vi "Main - network stream.vi"(8 "error in (no error)":T1) -> (0 "error out":T1)   [LabVIEW 2019, in "Communication Interface.lvlib"]
uses:
  Communication Interface.lvlib
  Intertarget communication/Status + response + data cluster.ctl
  module state.ctl
  module data.ctl
  Intertarget communication/CR_master_class/CR_master.lvclass
  Intertarget communication/CR slave_class/CR slave.lvclass
  5bf6cc24-2521-4779-a80f-885c0f377251.vi
  Intertarget communication/NS slave_class/NS slave.lvclass
  C:/Barkhausen mmWave radar/Development/modules/mmw_instrument/src_LabVIEW/Host/Intertarget communication/CR slave_class/CR slave.lvclass
  Intertarget communication/UE_master_class/UE_master.lvclass
  C:/Barkhausen mmWave radar/Development/modules/mmw_instrument/src_LabVIEW/Host/Intertarget communication/CR_master_class/CR_master.lvclass
  SubVIs/Shared/Comm GV.vi
  SubVIs/Shared/System GV.vi
  Intertarget communication/CommandResponse communication.lvlib
  SubVIs/Shared/Shared.lvlib
  ZMQ_mmWave_class/ZMQ_mmWave.lvclass
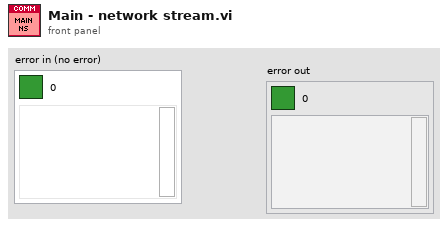
[diagram p1: front panel]
types:
  T1 = cluster{"Boolean Round":bool, "code":i32, "source":string}
  T2 = typedef "Communication Interface.lvlib/module state.ctl" = enum16{"init", "wait on connection", "communication", "close"}
  T3 = typedef "CommandResponse communication.lvlib/Status + response + data cluster.ctl" = cluster{"message":string, "response":string, "data":variant}
  T4 = typedef "Communication Interface.lvlib/module data.ctl" = cluster{"dummy":dbl, "HW Control":refnum<class "CR_master.lvclass">, "Command interface":refnum<class "CR slave.lvclass">}
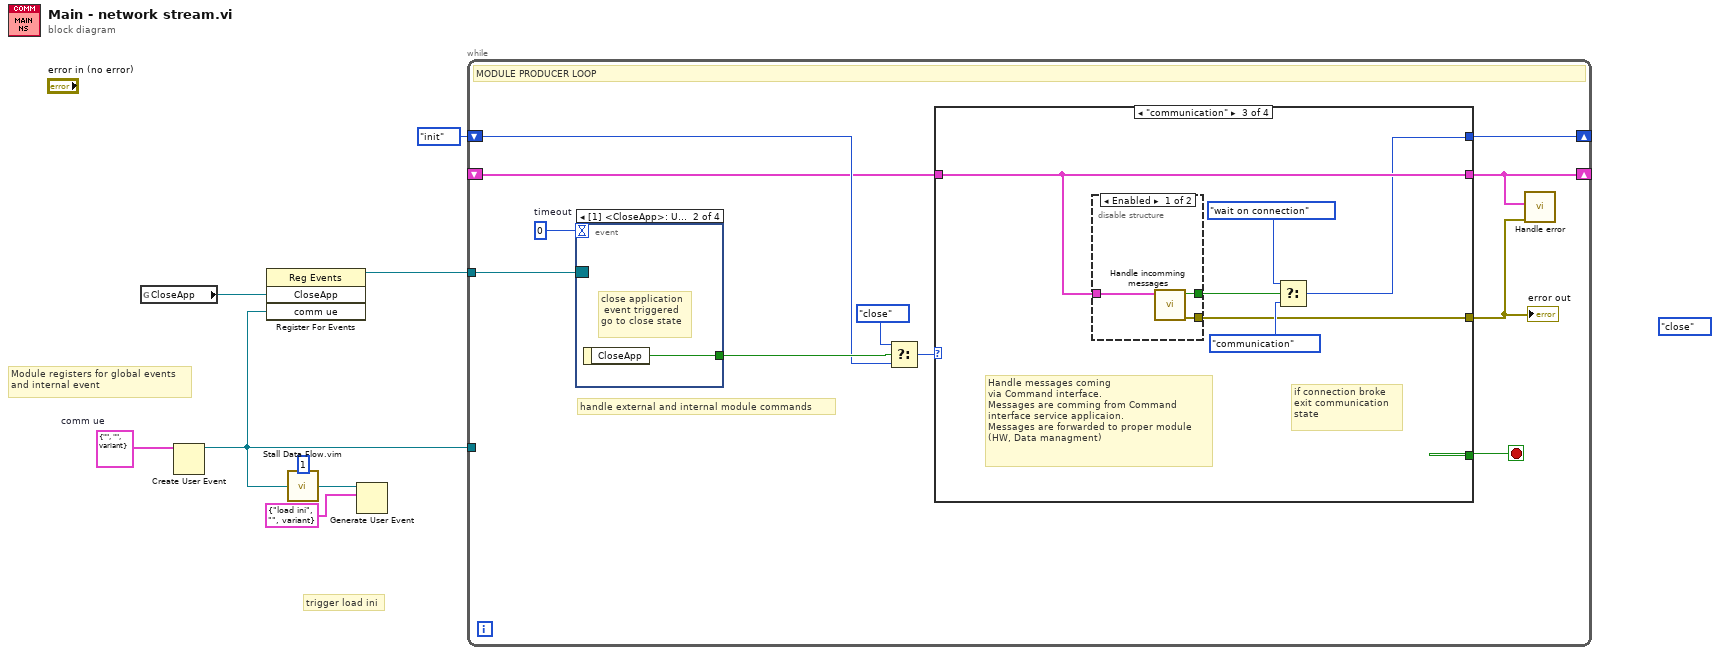
[diagram p0: block diagram]
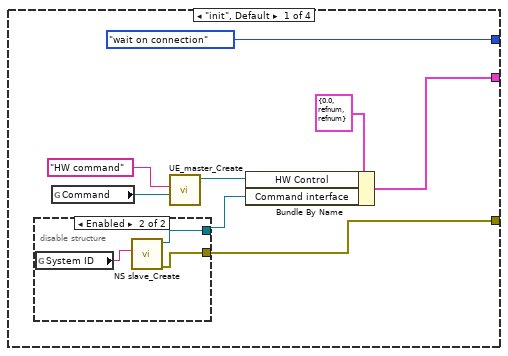
[diagram p2: hidden frame]
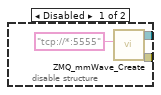
[diagram p3: hidden frame]
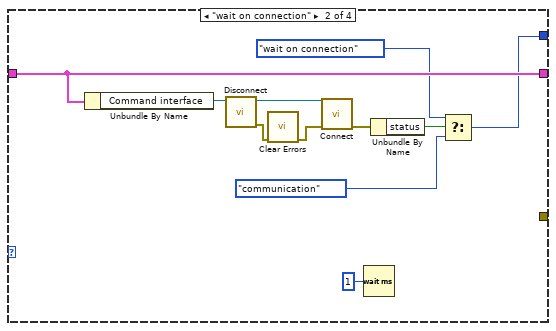
[diagram p4: hidden frame]
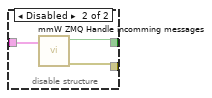
[diagram p5: hidden frame]
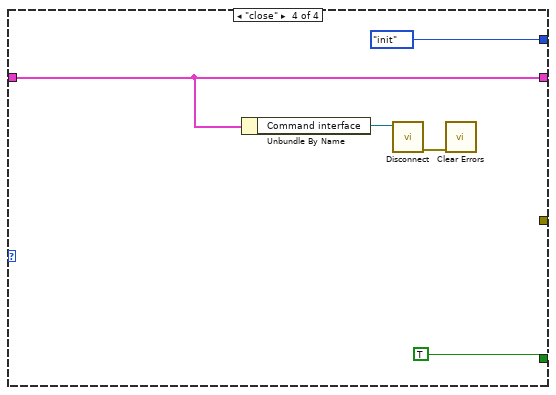
[diagram p6: hidden frame]
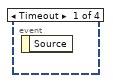
[diagram p7: hidden frame]
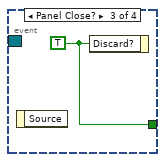
[diagram p8: hidden frame]
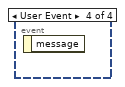
[diagram p9: hidden frame]
diagram:
  w4 = T3 {"message"="", "response"="", "data"=variant}  # comm ue
  (unwired) module_state."close" ("module states")
  # "trigger load ini"
  # "Module registers for global events\nand internal event"
  n1 = global read "Comm GV.vi" "CloseApp"() -> (w2:refnum<user-event>)
  n2 = Create User Event(user event datatype=w4) -> (user event=w7:refnum<user-event>)  [unwired: 1 in, 1 out]
  n3 = register-events(w2, w7) -> (reference out=w8:refnum<event-registration>)  [unwired: 2 in, 1 out]
  n4 = call "Stall Data Flow.vim"("value in"=w7, "milliseconds to wait"=u32 1) -> ("value out"=w6:refnum<user-event>)  [unwired: 1 out]
  n5 = Generate User Event(user event=w6, event data cluster=T3 {"message"="load ini", "response"="", "data"=variant} ("internal command")) -> ()  [unwired: 2 in, 2 out]
  n6 = while {
    tunnel: w8 -> [w19]
    tunnel: w7 -> [_]
    shift-right: [w11] -> _
    shift-left: _ -> [w12]
    shift-right: [w17] -> _
    shift-left: module_state."init" ("module states") -> [w15]
    stop <- w10 stop-if-true
    w18 = 0  # timeout
    # "handle external and internal module commands"
    # "MODULE PRODUCER LOOP"
    n7 = event shown="[1] <CloseApp>: User Event" {
      selector: w19 -> [_ _ _ _]
      dyn-events: _ -> [_ _ _ _]
      timeout: w18 -> [_ _ _ _]
      tunnel: [_ w62 w63 _] -> w16
      event Timeout {
        n8 = event-data() -> ()  [unwired: 1 in, 1 out]
      }
      event User Event {
        # "close application\n event triggered\ngo to close state"
        n9 = event-data() -> ("CloseApp"=w62:bool)  [unwired: 1 in]
      }
      event Panel Close? {
        w63 = TRUE ("Discard?")
        n10 = event-data() -> ()  [unwired: 1 in, 1 out]
        n11 = event-data("Discard?"=w63) -> ()  [unwired: 1 in, 1 out]
      }
      event User Event {
        n12 = event-data() -> ()  [unwired: 1 in, 1 out]
      }
    }
    n13 = Select(t=module_state."close", s=w16, f=w15) -> (s? t:f=w13:T2)
    n14 = case shown="\"communication\"" w13 {
      tunnel: [module_state."wait on connection" ("module states") w39 w47 module_state."init" ("t")] -> w17
      tunnel: [w21 w43 w50 w60] -> w11
      tunnel: w12 -> [_ w43 w50 w60]
      tunnel: [_ _ _ TRUE] -> w10
      tunnel: [w20 _ w45 _] -> w9
      frame "init", Default {
        n15 = disable-structure shown="Enabled" {
          disable-tunnel: [w29 w32] -> w26
          disable-tunnel: [w28 w31] -> w20
          frame Disabled {
            n16 = call "ZMQ_mmWave_Create.vi"("endpoint"="tcp://*:5555") -> ("error out"=w28:errorcluster, "reference out"=w29:refnum<class "ZMQ_mmWave.lvclass">)  [unwired: 9 in]
          }
          frame Enabled {
            n17 = global read "System GV.vi" "System ID"() -> (w33:string)
            n18 = call "NS slave_Create.vi"("ID"=w33) -> ("error out"=w31:errorcluster, "reference out"=w32:refnum<class "NS slave.lvclass">)  [unwired: 9 in]
          }
        }
        n19 = global read "Comm GV.vi" "Command"() -> (w23:refnum<user-event>)
        n20 = call "UE_master_Create.vi"("Command UE"=w23, "ID"="HW command") -> ("reference out"=w25:refnum<class "UE_master.lvclass">)  [unwired: 8 in, 1 out]
        n21 = Bundle By Name(cluster=T4 {"dummy"=0.0, "HW Control"=refnum, "Command interface"=refnum} ("module loopdata"), "HW Control"=w25, "Command interface"=w26) -> (w21:T4)
      }
      frame "wait on connection" {
        n22 = Unbundle By Name(w43) -> ("Command interface"=w42:refnum<class "CR slave.lvclass">)
        n23 = call-dynamic "Disconnect.vi"("reference in"=w42) -> ("error out"=w36:errorcluster, "reference out"=w37:refnum<class "CR slave.lvclass">)  [unwired: 9 in]
        n24 = call <vilib>:"Clear Errors.vi"("error in (no error)"=w36) -> ("error out"=w35:errorcluster)  [unwired: 5 in, 1 out]
        n25 = call-dynamic "Connect.vi"("error in (no error)"=w35, "reference in"=w37) -> ("error out"=w41:errorcluster)  [unwired: 8 in, 1 out]
        n26 = Wait (ms)(milliseconds to wait=u32 1) -> ()  [unwired: 1 out]
        n27 = Unbundle By Name(w41) -> ("status"=w40:bool)
        n28 = Select(t=module_state."wait on connection", s=w40, f=module_state."communication") -> (s? t:f=w39:T2)
      }
      frame "communication" {
        # "if connection broke\nexit communication\nstate"
        # "Handle messages coming\nvia Command interface.\nMessages are comming from Command\ninterface service applicaion.\nMessages are forwarded to proper module\n(HW, Data managment)"
        n29 = disable-structure shown="Enabled" {
          disable-tunnel: w50 -> [w53 w56]
          disable-tunnel: [w52 w55] -> w49
          disable-tunnel: [w51 w54] -> w45
          frame Enabled {
            n30 = call "Handle incomming messages.vi"("module loopdata"=w53) -> ("error out"=w51:errorcluster, "OK"=w52:bool)  [unwired: 9 in]
          }
          frame Disabled {
            n31 = call "mmW ZMQ Handle incomming messages.vi"("module loopdata"=w56) -> ("error out"=w54:errorcluster, "OK"=w55:bool)  [unwired: 9 in]
          }
        }
        n32 = Select(t=module_state."wait on connection", s=w49, f=module_state."communication" ("t")) -> (s? t:f=w47:T2)
      }
      frame "close" {
        n33 = Unbundle By Name(w60) -> ("Command interface"=w59:refnum<class "CR slave.lvclass">)
        n34 = call-dynamic "Disconnect.vi"("reference in"=w59) -> ("error out"=w57:errorcluster)  [unwired: 9 in, 1 out]
        n35 = call <vilib>:"Clear Errors.vi"("error in (no error)"=w57) -> ()  [unwired: 5 in, 2 out]
      }
    }
    "error out" <- w9
    n36 = call "Handle error.vi"("error in (no error)"=w9, "module loopdata"=w11) -> ()  [unwired: 9 in, 1 out]
  }
